vi "Set Tester Tx.vi"(8 "error in (no error)":errorcluster, 11 "Station Actor in":refnum<class "Station Actor.lvclass">) -> (0 "error out":errorcluster, 3 "Station Actor out":refnum<class "Station Actor.lvclass">)   [LabVIEW 2019, in "Station Actor.lvlib" / "Station Actor.lvclass"]
uses:
  Station Actor.lvclass
  Station Actor.lvclass/Station Actor.ctl
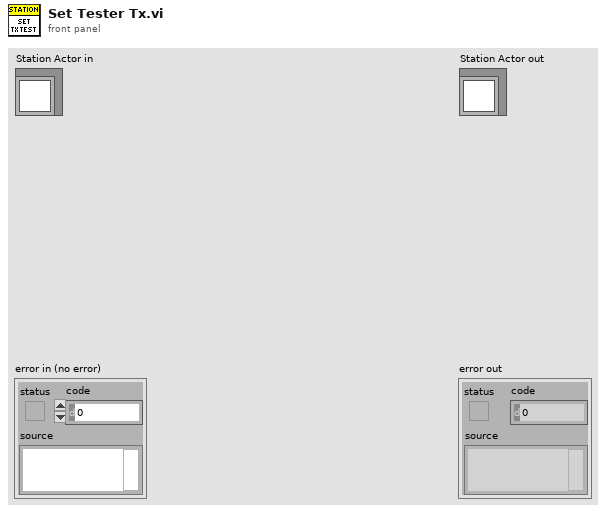
[diagram p1: front panel]
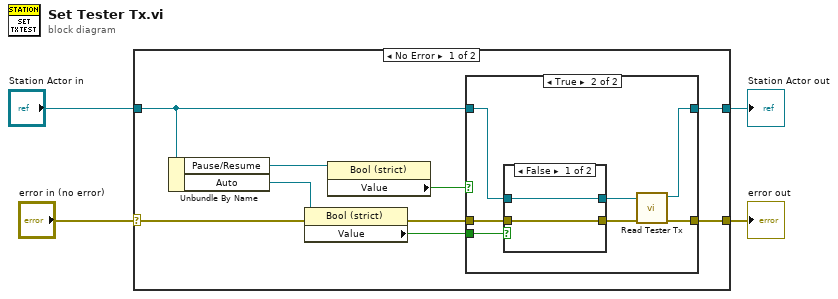
[diagram p0: block diagram]
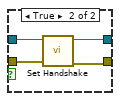
[diagram p3: hidden frame]
diagram:
  n1 = case shown="No Error" "error in (no error)" {
    selector: "error in (no error)" -> [w8 w30]
    tunnel: [w13 w30] -> w3
    tunnel: [w5 w29] -> w1
    tunnel: "Station Actor in" -> [w6 w29]
    frame No Error {
      n2 = Unbundle By Name(w6) -> ("Pause/Resume"=w12:refnum<vi>, "Auto"=w10:refnum<vi>)
      n3 = property class="Bool (strict)"(reference=w10, error in=w8) -> (error out=w7:errorcluster, "Value"=w9:bool)  [unwired: 1 out]
      n4 = property class="Bool (strict)"(reference=w12) -> ("Value"=w11:bool)  [unwired: 1 in, 2 out]
      n5 = case shown="True" w11 {
        tunnel: w7 -> [w15 w22]
        tunnel: [w15 w19] -> w13
        tunnel: w9 -> [_ w21]
        tunnel: w6 -> [w14 w17]
        tunnel: [w14 w18] -> w5
        frame False {
        }
        frame True {
          n6 = case shown="False" w21 {
            tunnel: w22 -> [w24 w28]
            tunnel: [w24 w27] -> w20
            tunnel: w17 -> [w23 w26]
            tunnel: [w23 w25] -> w16
            frame False {
            }
            frame True {
              n7 = call "Set Handshake.vi"("error in (no error)"=w28, "Panel in"=w26) -> ("error out"=w27:errorcluster, "Panel out"=w25:refnum<class "Station Actor.lvclass">)  [unwired: 8 in]
            }
          }
          n8 = call "Read Tester Tx.vi"("error in (no error)"=w20, "Panel in"=w16) -> ("error out"=w19:errorcluster, "Panel out"=w18:refnum<class "Station Actor.lvclass">)  [unwired: 8 in]
        }
      }
    }
    frame Error {
    }
  }
  "error out" <- w3
  "Station Actor out" <- w1
